vi "Get Id.vi"(7 "error in (no error)":errorcluster, 10 "Instrument Name":string) -> (0 "error out":errorcluster, 2 "ID of IDN Command":string, 3 "CommandDirectors":refnum<class "CommandDirector.lvclass">[](array[class]))   [LabVIEW 2023]
doc: "Asks the framework to run a *IDN? command on the passed Instrument. The framework will turn the Instrument Name into an actual Driver instance, set up the Command and Command Director and get a Test Processor to actually run the command. Note that the result isn't returned through this VI but through the Results Notifier."
uses:
  CommandDirector/CommandDirector.lvclass
  ResourceEnumerator/ResourceEnumerator.lvclass
  RST/RST.lvclass
  \\Mac\Home/Documents/LabVIEW Data/ProjectTemplates/Source/HAF/WriteCommand/WriteCommand.lvclass
  IDN/IDN.lvclass
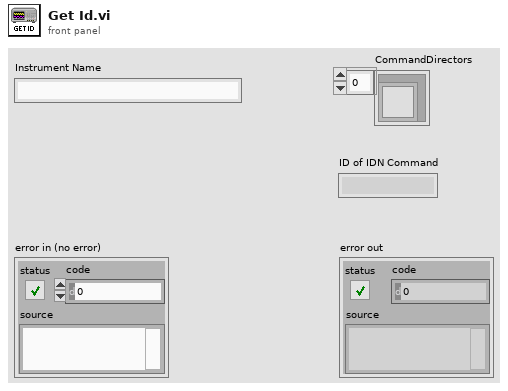
[diagram p1: front panel]
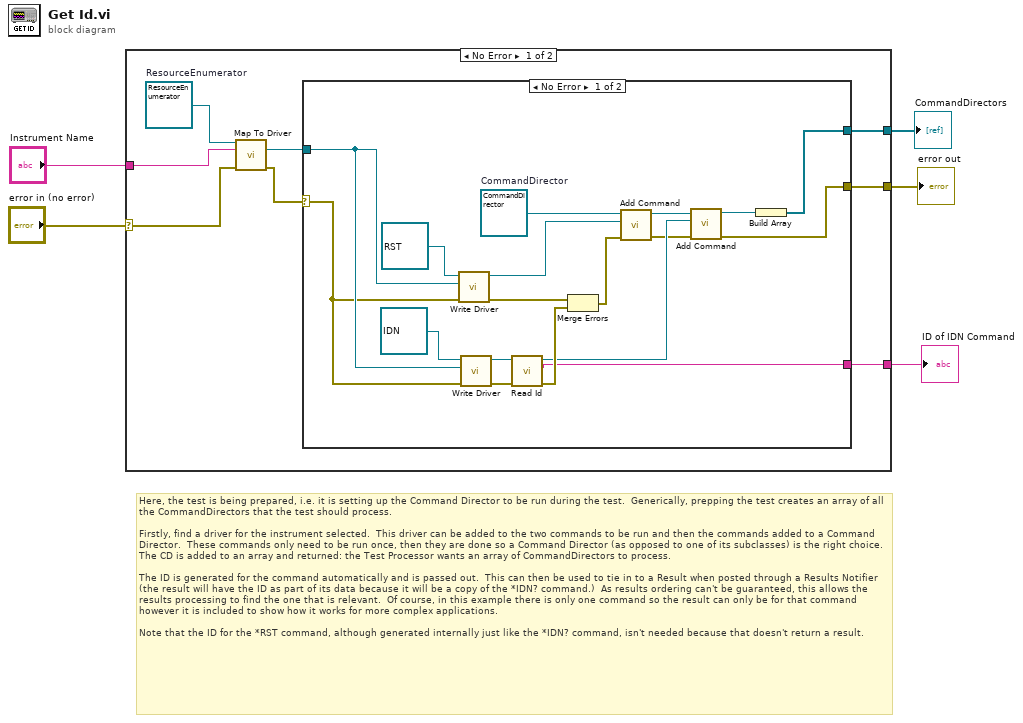
[diagram p0: block diagram]
diagram:
  # "Here, the test is being prepared, i.e. it is setting up the Command Director to be run during the test.  Generically, prepping the test creates an array of all the CommandDirectors that the test should process.  \n\nFirstly, find a driver for the instrument selected.  This driver can be added to the two commands to be run and then the commands added to a Command Director.  These commands only need to be run once, then they are done so a Command Director (as opposed to one of its subclasses) is the right choice.  The CD is added to an array and returned: the Test Processor wants an array of CommandDirectors to process.\n\nThe ID is generated for the command automatically and is passed out.  This can then be used to tie in to a Result when posted through a Results Notifier (the result will have the ID as part of its data because it will be a copy of the *IDN? command.)  As results ordering can't be guaranteed, this allows the results processing to find the one that is relevant.  Of course, in this example there is only one command so the result can only be for that command however it is included to show how it works for more complex applications.\n\nNote that the ID for the *RST command, although generated internally just like the *IDN? command, isn't needed because that doesn't return a result."
  n1 = case shown="No Error" "error in (no error)" {
    selector: "error in (no error)" -> [w12 w33]
    tunnel: "Instrument Name" -> [w11 _]
    tunnel: [w8 _] -> w2
    tunnel: [w7 w33] -> w3
    tunnel: [w6 _] -> w1
    frame No Error {
      w13 = refnum<class "ResourceEnumerator.lvclass"> refnum  # ResourceEnumerator
      n2 = call-dynamic "Map To Driver.vi"("AbstractResourceEnumerator in"=w13, "Driver Name"=w11, "error in (no error)"=w12) -> ("Driver"=w9:refnum<class "Driver.lvclass">, "error out"=w10:errorcluster)  [unwired: 10 in, 1 out]
      n3 = case shown="No Error" w10 {
        selector: w10 -> [w28 w32]
        tunnel: w9 -> [w29 _]
        tunnel: [w17 _] -> w8
        tunnel: [w14 w32] -> w7
        tunnel: [w15 _] -> w6
        frame No Error {
          w26 = refnum<class "CommandDirector.lvclass"> refnum  # CommandDirector
          n4 = call-dynamic "Write Driver.vi"("error in (no error)"=w28, "HAF:Driver.lvclass"=w29, "WriteCommand in"=refnum<class "RST.lvclass"> refnum ("HAF:RST.lvclass")) -> ("error out"=w27:errorcluster, "WriteCommand out"=w25:refnum<class "RST.lvclass">)  [unwired: 7 in]
          n5 = call-dynamic "Write Driver.vi"("error in (no error)"=w28, "HAF:Driver.lvclass"=w29, "WriteCommand in"=refnum<class "IDN.lvclass"> refnum ("HAF:IDN.lvclass")) -> ("error out"=w22:errorcluster, "WriteCommand out"=w23:refnum<class "IDN.lvclass">)  [unwired: 7 in]
          n6 = call-dynamic "Read Id.vi"("error in (no error)"=w22, "WriteCommand in"=w23) -> ("error out"=w21:errorcluster, "Id"=w17:string, "WriteCommand out"=w19:refnum<class "IDN.lvclass">)  [unwired: 7 in]
          n7 = Merge Errors(w27, w21) -> (w24:errorcluster)
          n8 = call-dynamic "Add Command.vi"("error in (no error)"=w24, "Write Command"=w25, "Command Director in"=w26) -> ("error out"=w18:errorcluster, "Command Director out"=w20:refnum<class "CommandDirector.lvclass">)  [unwired: 7 in]
          n9 = call-dynamic "Add Command.vi"("error in (no error)"=w18, "Write Command"=w19, "Command Director in"=w20) -> ("error out"=w14:errorcluster, "Command Director out"=w16:refnum<class "CommandDirector.lvclass">)  [unwired: 7 in]
          n10 = Build Array(w16) -> (w15:refnum<class "CommandDirector.lvclass">[])
        }
        frame Error {
        }
      }
    }
    frame Error {
    }
  }
  "error out" <- w3
  "ID of IDN Command" <- w2
  "CommandDirectors" <- w1
